vi "GEA3 HEWH Standard ERD List.vi"(8 "Error In":errorcluster) -> (0 "Error Out":errorcluster, 2 "Header":string[](array[string]), 3 "Read ERD List":T1[](array[typedef]) {"ERD Number" format="%.0x"})   [LabVIEW 2016]
uses:
  type defs/ERD Read Data In.ctl
  type defs/Data Type.ctl
  <vilib>/Utility/error.llb/whitespace.ctl
  library/GEA2_Toolkit.lvlib
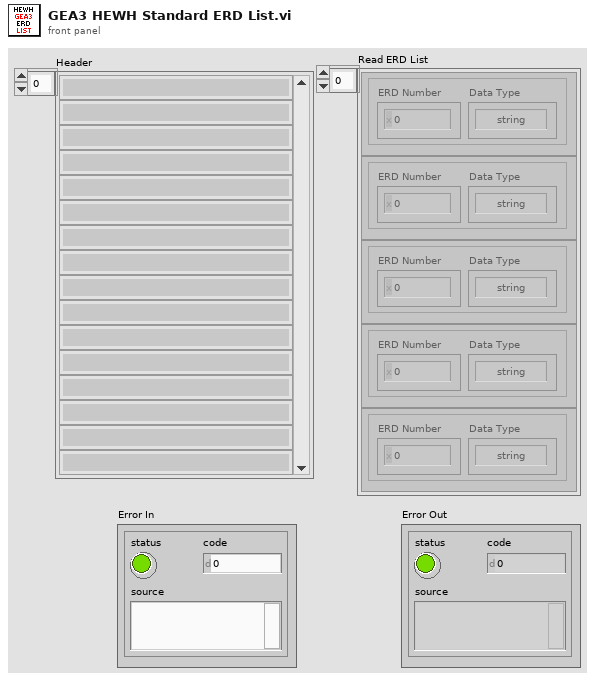
[diagram p1: front panel]
types:
  T1 = typedef "GEA2_Toolkit.lvlib/ERD Read Data In.ctl" = cluster{"ERD Number":u16, "Data Type":T2}
  T2 = typedef "GEA2_Toolkit.lvlib/Data Type.ctl" = enum16{"string", "boolean", "uint8_t", "uint16_t", "uint32_t", "uint64_t", "int8_t", "int16_t", "int32_t", "int64_t"}
  T3 = typedef "whitespace.ctl" = u16
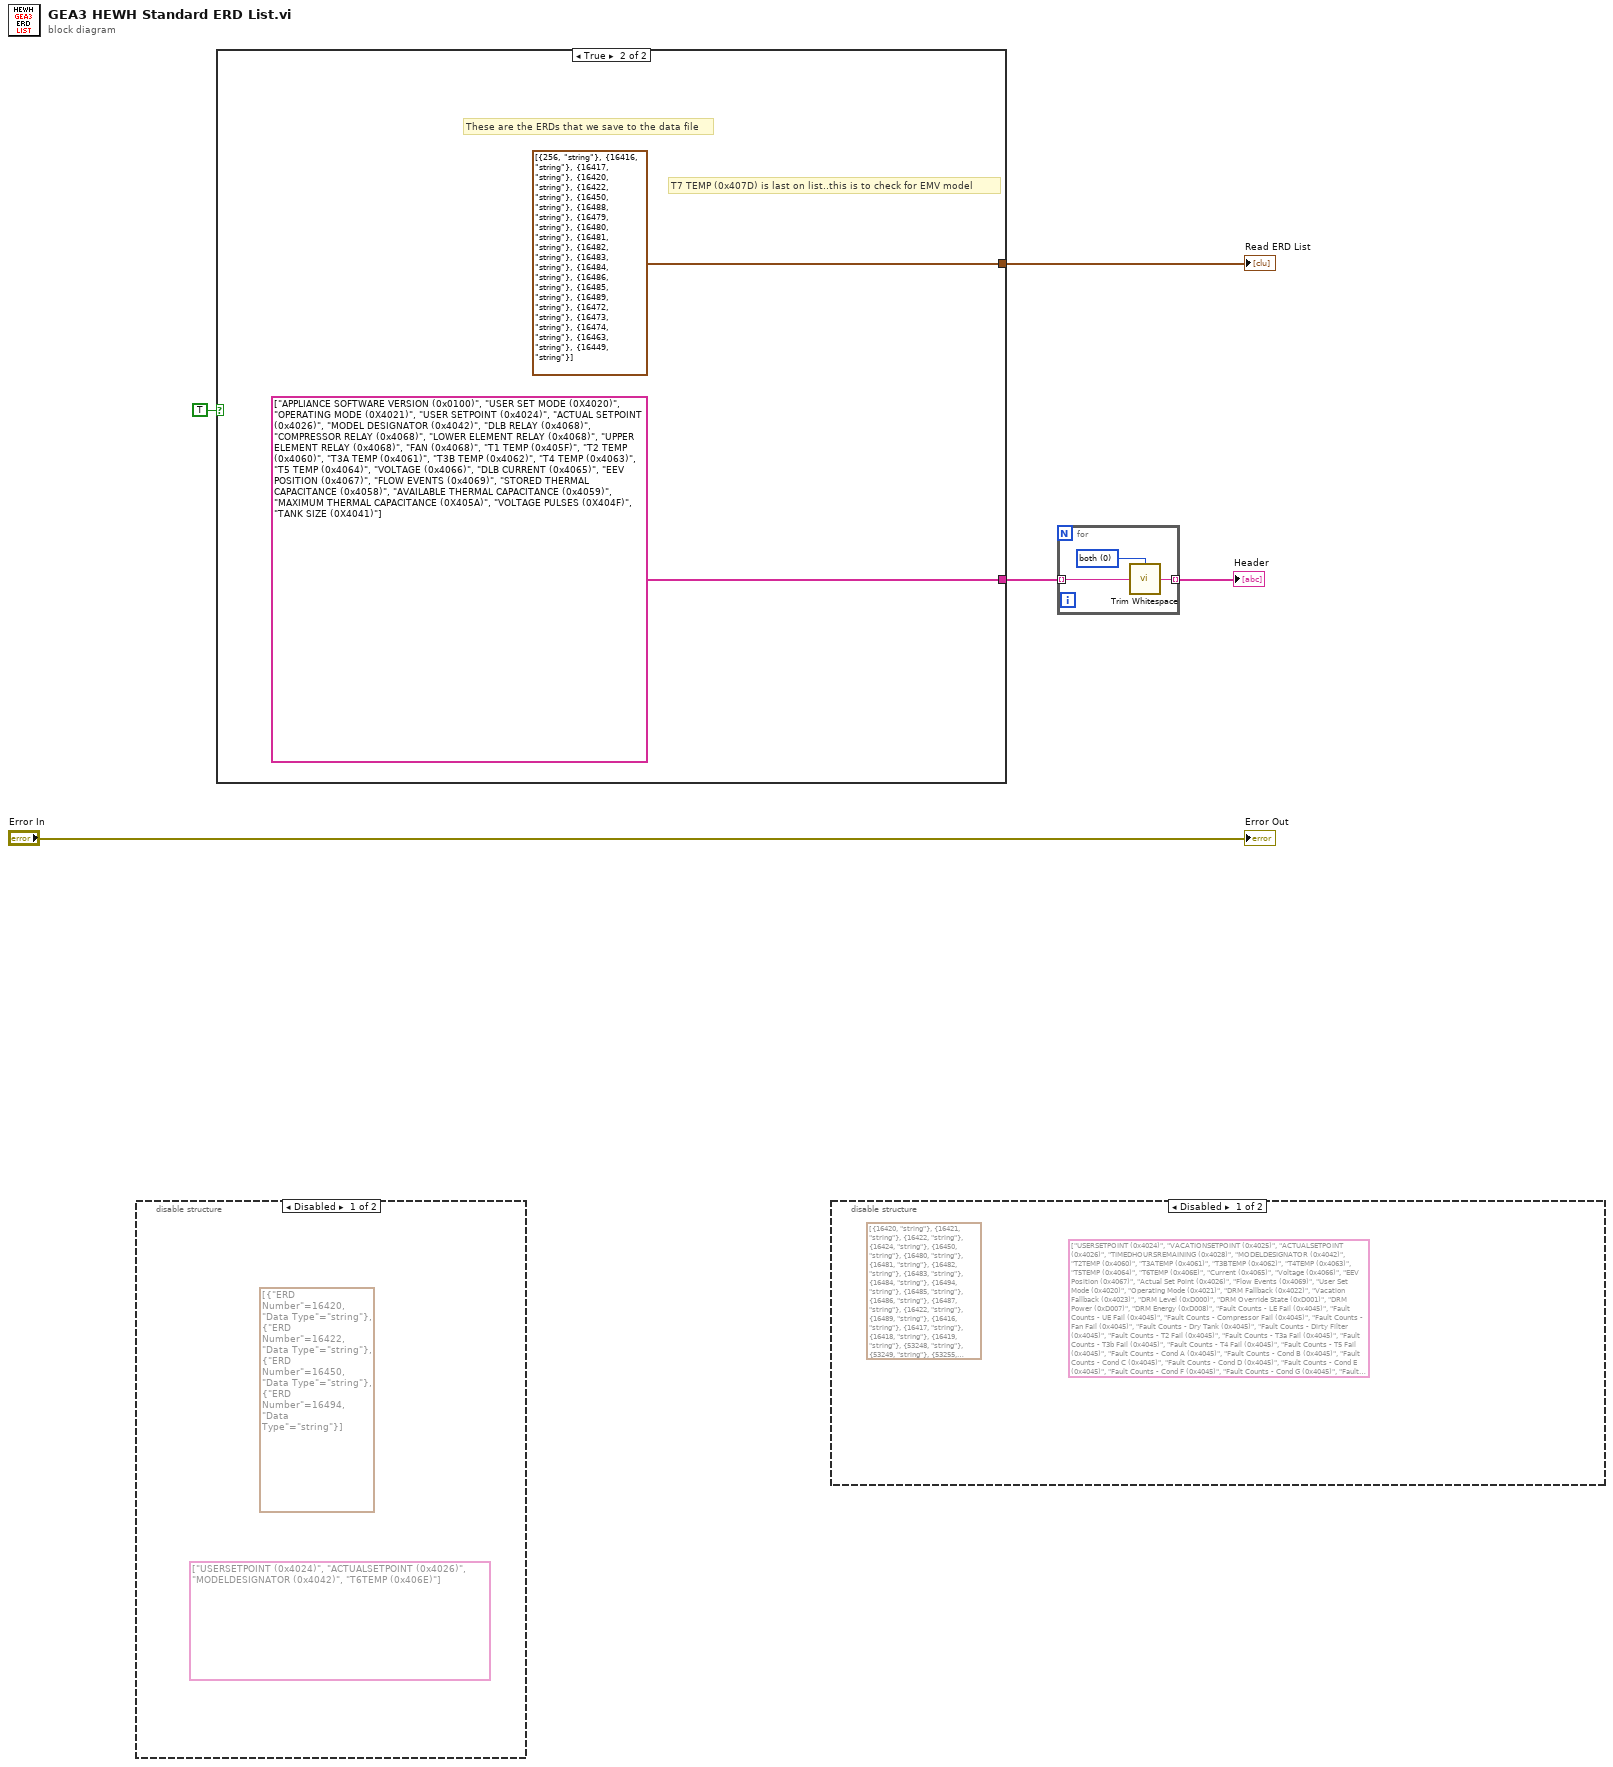
[diagram p0: block diagram]
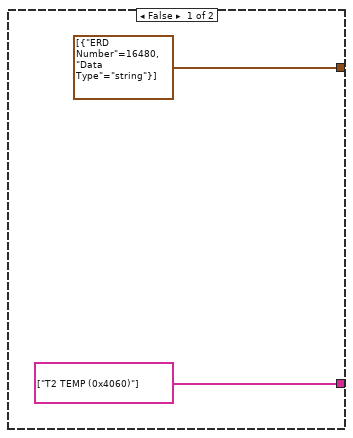
[diagram p2: hidden frame]
diagram:
  n1 = disable-structure shown="Disabled" {
    frame Disabled {
      (unwired) string[] ["USERSETPOINT (0x4024)", "ACTUALSETPOINT (0x4026)", "MODELDESIGNATOR (0x4042)", "T6TEMP (0x406E)"]
      (unwired) T1[] [{"ERD Number"=16420, "Data Type"=enum."string"}, {"ERD Number"=16422, "Data Type"=enum."string"}, {"ERD Number"=16450, "Data Type"=enum."string"}, {"ERD Number"=16494, "Data Type"=enum."string"}] ("Read ERD List")
    }
    frame Enabled {
    }
  }
  n2 = case shown="True" TRUE {
    tunnel: [T1[] [{"ERD Number"=16480, "Data Type"=enum."string"}] ("Read ERD List") T1[] [{"ERD Number"=256, "Data Type"=enum."string"}, {"ERD Number"=16416, "Data Type"=enum."string"}, {"ERD Number"=16417, "Data Type"=enum."string"}, {"ERD Number"=16420, "Data Type"=enum."string"}, {"ERD Number"=16422, "Data Type"=enum."string"}, {"ERD Number"=16450, "Data Type"=enum."string"}, {"ERD Number"=16488, "Data Type"=enum."string"}, {"ERD Number"=16479, "Data Type"=enum."string"}, {"ERD Number"=16480, "Data Type"=enum."string"}, {"ERD Number"=16481, "Data Type"=enum."string"}, {"ERD Number"=16482, "Data Type"=enum."string"}, {"ERD Number"=16483, "Data Type"=enum."string"}, {"ERD Number"=16484, "Data Type"=enum."string"}, {"ERD Number"=16486, "Data Type"=enum."string"}, {"ERD Number"=16485, "Data Type"=enum."string"}, {"ERD Number"=16489, "Data Type"=enum."string"}, {"ERD Number"=16472, "Data Type"=enum."string"}, {"ERD Number"=16473, "Data Type"=enum."string"}, {"ERD Number"=16474, "Data Type"=enum."string"}, {"ERD Number"=16463, "Data Type"=enum."string"}, {"ERD Number"=16449, "Data Type"=enum."string"}] ("Read ERD List")] -> w5
    tunnel: [string[] ["T2 TEMP (0x4060)"] string[] ["APPLIANCE SOFTWARE VERSION (0x0100)", "USER SET MODE (0X4020)", "OPERATING MODE (0X4021)", "USER SETPOINT (0x4024)", "ACTUAL SETPOINT (0x4026)", "MODEL DESIGNATOR (0x4042)", "DLB RELAY (0x4068)", "COMPRESSOR RELAY (0x4068)", "LOWER ELEMENT RELAY (0x4068)", "UPPER ELEMENT RELAY (0x4068)", "FAN (0x4068)", "T1 TEMP (0x405F)", "T2 TEMP (0x4060)", "T3A TEMP (0x4061)", "T3B TEMP (0x4062)", "T4 TEMP (0x4063)", "T5 TEMP (0x4064)", "VOLTAGE (0x4066)", "DLB CURRENT (0x4065)", "EEV POSITION (0x4067)", "FLOW EVENTS (0x4069)", "STORED THERMAL CAPACITANCE (0x4058)", "AVAILABLE THERMAL CAPACITANCE (0x4059)", "MAXIMUM THERMAL CAPACITANCE (0X405A)", "VOLTAGE PULSES (0X404F)", "TANK SIZE (0X4041)"]] -> w2
    frame False {
    }
    frame True {
      # "T7 TEMP (0x407D) is last on list..this is to check for EMV model"
      # "These are the ERDs that we save to the data file"
    }
  }
  "Read ERD List" <- w5
  n3 = disable-structure shown="Disabled" {
    frame Disabled {
      (unwired) string[] ["USERSETPOINT (0x4024)", "VACATIONSETPOINT (0x4025)", "ACTUALSETPOINT (0x4026)", "TIMEDHOURSREMAINING (0x4028)", "MODELDESIGNATOR (0x4042)", "T2TEMP (0x4060)", "T3ATEMP (0x4061)", "T3BTEMP (0x4062)", "T4TEMP (0x4063)", "T5TEMP (0x4064)", "T6TEMP (0x406E)", "Current (0x4065)", "Voltage (0x4066)", "EEV Position (0x4067)", "Actual Set Point (0x4026)", "Flow Events (0x4069)", "User Set Mode (0x4020)", "Operating Mode (0x4021)", "DRM Fallback (0x4022)", "Vacation Fallback (0x4023)", "DRM Level (0xD000)", "DRM Override State (0xD001)", "DRM Power (0xD007)", "DRM Energy (0xD008)", "Fault Counts - LE Fail (0x4045)", "Fault Counts - UE Fail (0x4045)", "Fault Counts - Compressor Fail (0x4045)", "Fault Counts - Fan Fail (0x4045)", "Fault Counts - Dry Tank (0x4045)", "Fault Counts - Dirty Filter (0x4045)", "Fault Counts - T2 Fail (0x4045)", "Fault Counts - T3a Fail (0x4045)", "Fault Counts - T3b Fail (0x4045)", "Fault Counts - T4 Fail (0x4045)", "Fault Counts - T5 Fail (0x4045)", "Fault Counts - Cond A (0x4045)", "Fault Counts - Cond B (0x4045)", "Fault Counts - Cond C (0x4045)", "Fault Counts - Cond D (0x4045)", "Fault Counts - Cond E (0x4045)", "Fault Counts - Cond F (0x4045)", "Fault Counts - Cond G (0x4045)", "Fault Counts - Cond H (0x4045)", "Fault Counts - Cond I (0x4045)", "Fault Counts - Cond J (0x4045)", "Fault Counts - Cond L (0x4045)", "Condensate Drain Pan Voltage (0x4071)", "Relay States - DLB (0x4068)", "Relay States - Compressor (0x4068)", "Relay States - Upper Element (0x4068)", "Relay States - Lower Element (0x4068)", "Relay States - Fan (0x4068)", "Compressor Min On/Off Time (0x406B)", "SS Run State (0x406C)"]
      (unwired) T1[] [{"ERD Number"=16420, "Data Type"=enum."string"}, {"ERD Number"=16421, "Data Type"=enum."string"}, {"ERD Number"=16422, "Data Type"=enum."string"}, {"ERD Number"=16424, "Data Type"=enum."string"}, {"ERD Number"=16450, "Data Type"=enum."string"}, {"ERD Number"=16480, "Data Type"=enum."string"}, {"ERD Number"=16481, "Data Type"=enum."string"}, {"ERD Number"=16482, "Data Type"=enum."string"}, {"ERD Number"=16483, "Data Type"=enum."string"}, {"ERD Number"=16484, "Data Type"=enum."string"}, {"ERD Number"=16494, "Data Type"=enum."string"}, {"ERD Number"=16485, "Data Type"=enum."string"}, {"ERD Number"=16486, "Data Type"=enum."string"}, {"ERD Number"=16487, "Data Type"=enum."string"}, {"ERD Number"=16422, "Data Type"=enum."string"}, {"ERD Number"=16489, "Data Type"=enum."string"}, {"ERD Number"=16416, "Data Type"=enum."string"}, {"ERD Number"=16417, "Data Type"=enum."string"}, {"ERD Number"=16418, "Data Type"=enum."string"}, {"ERD Number"=16419, "Data Type"=enum."string"}, {"ERD Number"=53248, "Data Type"=enum."string"}, {"ERD Number"=53249, "Data Type"=enum."string"}, {"ERD Number"=53255, "Data Type"=enum."string"}, {"ERD Number"=53256, "Data Type"=enum."string"}, {"ERD Number"=16453, "Data Type"=enum."string"}, {"ERD Number"=16497, "Data Type"=enum."string"}, {"ERD Number"=16488, "Data Type"=enum."string"}, {"ERD Number"=16491, "Data Type"=enum."string"}, {"ERD Number"=16492, "Data Type"=enum."string"}] ("Read ERD List")
    }
    frame Enabled {
    }
  }
  n4 = for {
    tunnel: w2 -> [w11] mode=indexing
    tunnel: [w10] -> w3 mode=indexing
    w12 = T3 0 items=["both", "start of string", "end of string"] ("location (both)")
    n5 = call <vilib>:"Trim Whitespace.vi"("string"=w11, "location (both)"=w12) -> ("trimmed string"=w10:string)
  }
  "Header" <- w3
  "Error Out" <- "Error In"
